vi "Teleop.vi"(10 "Match Info":T1={"Autonomous Elapsed Seconds"=0.0, "TeleOp Elapsed Seconds"=0.0, "Disabled Elapsed Seconds"=0.0, "Visited Autonomous"=FALSE, "Visited TeleOp"=FALSE, "Visited Disabled"=FALSE, "Autonomous Settings"={"Autonomous Style"=enum."Independent", "VI Refnum"=refnum}}, 11 "Call Context":T2) -> ()   [LabVIEW 2020]
doc: "This VI is called for each TeleOp packet received from the DS where the robot is not disabled. It is often used to read from the joysticks and update I/O or to update setpoints for timed control loops. It should complete and return within 20 milliseconds or it may miss DS packets."
uses:
  <vilib>/Rock Robotics/WPI/DriverStation/WPI_DriverStationDerivedRobotMode.ctl
  <vilib>/Rock Robotics/WPI/DriverStation/WPI_DriverStationMatch Info.ctl
  <vilib>/Rock Robotics/WPI/Utilities/WPI_GetSetVariantRefNum.vi
  2017 Swerve Code/Swerve Global Variables.vi
  Robot Global Data.vi
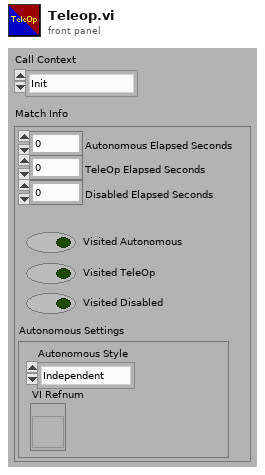
[diagram p1: front panel]
types:
  T1 = typedef "WPI_DriverStationMatch Info.ctl" = cluster{"Autonomous Elapsed Seconds":dbl, "TeleOp Elapsed Seconds":dbl, "Disabled Elapsed Seconds":dbl, "Visited Autonomous":bool, "Visited TeleOp":bool, "Visited Disabled":bool, "Autonomous Settings":cluster{"Autonomous Style":enum16{"Iterative", "Independent"}, "VI Refnum":refnum<vi>}}
  T2 = typedef "WPI_DriverStationDerivedRobotMode.ctl" = enum16{"Init", "Execute", "Stop"}
  T3 = typedef "WPI_JoystickDevRef.ctl" = cluster{"Device":T4}
  T4 = typedef "WPI_JoystickDeviceEnum.ctl" = enum16{"USB 0", "USB 1", "USB 2", "USB 3", "USB 4", "USB 5"}
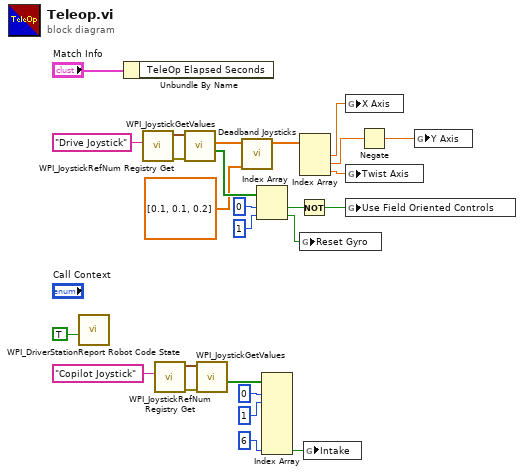
[diagram p0: block diagram]
diagram:
  n1 = call <vilib>:"WPI_DriverStationReport Robot Code State.vi"("TeleOp"=TRUE ("Autonomous")) -> ()  [unwired: 10 in, 1 out]
  n2 = Unbundle By Name("Match Info") -> ()  [unwired: 1 out]
  n3 = call <vilib>:"WPI_JoystickRefNum Registry Get.vi"("refnum name"="Drive Joystick") -> ("error out"=w14:errorcluster, "JoystickDevRef"=w24:T3)  [unwired: 1 in, 8 out]
  n4 = call <vilib>:"WPI_JoystickRefNum Registry Get.vi"("refnum name"="Copilot Joystick") -> ("error out"=w8:errorcluster, "JoystickDevRef"=w9:T3)  [unwired: 1 in, 8 out]
  n5 = call <vilib>:"WPI_JoystickGetValues.vi"("error in (no error)"=w14, "JoystickDevRef"=w24) -> ("Buttons"=w18:bool[], "Axes"=w13:dbl[])  [unwired: 5 in, 3 out]
  n6 = call <vilib>:"WPI_JoystickGetValues.vi"("error in (no error)"=w8, "JoystickDevRef"=w9) -> ("Buttons"=w7:bool[])  [unwired: 5 in, 4 out]
  n7 = call "Deadband Joysticks.vi"("Deadbands"=dbl[] [0.1, 0.1, 0.2], "Axes"=w13) -> ("Axes'"=w11:dbl[])  [unwired: 9 in]
  n8 = Index Array(array=w18, index #1=0 ("index"), index #2=1 ("index")) -> (element #1=w17:bool, element #2=w15:bool)
  n9 = Index Array(array=w7, index #1=0 ("index"), index #2=1 ("index"), index #8=6 ("index")) -> (element #8=w1:bool)  [unwired: 5 in, 7 out]
  n10 = Not(x=w17) -> (.not. x?=w16:bool)
  n11 = Index Array(array=w11) -> (element #1=w22:dbl, element #2=w21:dbl, element #3=w20:dbl)  [unwired: 3 in]
  n12 = global write "Swerve Global Variables.vi" "Reset Gyro"(w15) -> ()
  n13 = global write "Robot Global Data.vi" "Intake"(w1) -> ()
  n14 = global write "Swerve Global Variables.vi" "X Axis"(w22) -> ()
  n15 = global write "Swerve Global Variables.vi" "Twist Axis"(w20) -> ()
  n16 = global write "Swerve Global Variables.vi" "Use Field Oriented Controls"(w16) -> ()
  n17 = Negate(x=w21) -> (-x=w19:dbl)
  n18 = global write "Swerve Global Variables.vi" "Y Axis"(w19) -> ()
